vi "CH2_Rx.vi"() -> ()   [LabVIEW 2018]
uses:
  Stream/Stream.lvclass
  RxTx/RxTx.lvclass
  Stream/Stream.lvclass/Stream.ctl
panel:
  in  "RxTx.lvclass":refnum<class "RxTx.lvclass">
  in  "Stream.lvclass":refnum<class "Stream.lvclass">
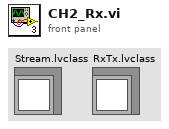
[diagram p1: front panel]
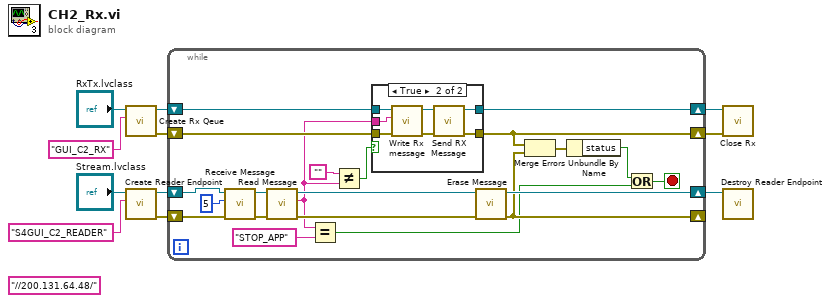
[diagram p0: block diagram]
diagram:
  (unwired) "//200.131.64.48/" ("Reader Name")
  n1 = call "Create Rx Qeue.vi"("Reader Name"="GUI_C2_RX", "RxTx in"="RxTx.lvclass") -> ("error out"=w4:errorcluster, "RxTx out"=w5:refnum<class "RxTx.lvclass">)  [unwired: 8 in]
  n2 = call "Create Reader Endpoint.vi"("reader name"="S4GUI_C2_READER", "Stream in"="Stream.lvclass") -> ("error out"=w9:errorcluster, "Stream out"=w10:refnum<class "Stream.lvclass">)  [unwired: 8 in]
  n3 = while {
    shift-right: [w18] -> _
    shift-left: w9 -> [w31]
    shift-right: [w21] -> w8
    shift-left: w10 -> [w32]
    shift-right: [w25] -> w2
    shift-left: w4 -> [w28]
    shift-right: [w27] -> w3
    shift-left: w5 -> [w13]
    stop <- w16 stop-if-true
    n4 = call "Receive Message.vi"("error in (no error)"=w31, "timeout ms"=5, "Stream in"=w32) -> ("error out"=w29:errorcluster, "Stream out"=w30:refnum<class "Stream.lvclass">)  [unwired: 7 in]
    n5 = call "Read Message.vi"("error in (no error)"=w29, "Stream in"=w30) -> ("error out"=w20:errorcluster, "Message"=w12:string, "Stream out"=w19:refnum<class "Stream.lvclass">)  [unwired: 7 in]
    n6 = Equal?(x=w12, y="STOP_APP" ("reader name")) -> (x = y?=w14:bool)
    n7 = Not Equal?(x="", y=w12) -> (x != y?=w22:bool)
    n8 = case shown="True" w22 {
      tunnel: w28 -> [w33 w39]
      tunnel: w13 -> [w34 w38]
      tunnel: w12 -> [_ w37]
      tunnel: [w34 w36] -> w27
      tunnel: [w33 w35] -> w25
      frame False {
      }
      frame True {
        n9 = call "Write Rx message.vi"("error in (no error)"=w39, "Rx message"=w37, "RxTx in"=w38) -> ("error out"=w40:errorcluster, "RxTx out"=w41:refnum<class "RxTx.lvclass">)  [unwired: 7 in]
        n10 = call "Send RX Message.vi"("error in (no error)"=w40, "RxTx in"=w41) -> ("error out"=w35:errorcluster, "RxTx out"=w36:refnum<class "RxTx.lvclass">)  [unwired: 8 in]
      }
    }
    n11 = call "Erase Message.vi"("error in (no error)"=w20, "Stream in"=w19) -> ("error out"=w18:errorcluster, "Stream out"=w21:refnum<class "Stream.lvclass">)  [unwired: 8 in]
    n12 = Merge Errors(w25, w18) -> (w26:errorcluster)
    n13 = Unbundle By Name(w26) -> ("status"=w15:bool)
    n14 = Or(x=w15, y=w14) -> (x .or. y?=w16:bool)
  }
  n15 = call "Close Rx.vi"("error in (no error)"=w2, "RxTx in"=w3) -> ()  [unwired: 8 in, 2 out]
  n16 = call "Destroy Reader Endpoint.vi"("Stream in"=w8) -> ()  [unwired: 9 in, 2 out]
